vi "Encoder.vi"(11 "Frequency":dbl) -> (1 "Encoder Position (mm)":dbl[](array[numeric]), 2 "RPM":dbl[](array[numeric])=[1.7549382010467513e-60, 1.807415273169756e-52])   [LabVIEW 2021]
uses:
  <vilib>/Analysis/3filter.llb/Filter Passband Type.ctl
  <vilib>/ptbypt/NI_PtbyPt.lvlib
  <vilib>/Analysis/NI_AALBase.lvlib
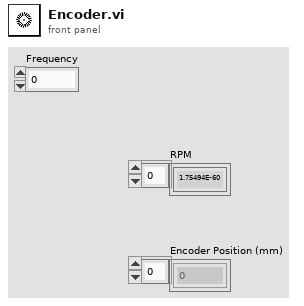
[diagram p1: front panel]
types:
  T1 = typedef "NI_AALBase.lvlib/Filter Passband Type.ctl" = enum32{"Lowpass", "Highpass", "Bandpass", "Bandstop"}
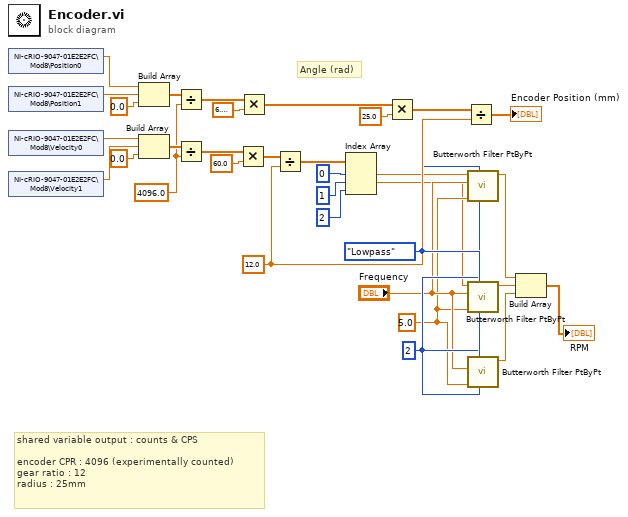
[diagram p0: block diagram]
diagram:
  w19 = 12.0 ("y")
  w23 = 4096.0 ("y")
  w13 = 2 ("order")
  w11 = 5.0 ("low cutoff freq: fl")
  w14 = Filter_Passband_Type."Lowpass" ("filter type")
  # "Angle (rad)"
  # "shared variable output : counts & CPS\n\nencoder CPR : 4096 (experimentally counted)\ngear ratio : 12\nradius : 25mm"
  n1 = shared-variable "NI-cRIO-9047-01E2E2FC\\Mod8\\Position0"() -> (w27:dbl)  [unwired: 1 in, 1 out]
  n2 = shared-variable "NI-cRIO-9047-01E2E2FC\\Mod8\\Position1"() -> (w26:dbl)  [unwired: 1 in, 1 out]
  n3 = shared-variable "NI-cRIO-9047-01E2E2FC\\Mod8\\Velocity0"() -> (w31:dbl)  [unwired: 1 in, 1 out]
  n4 = shared-variable "NI-cRIO-9047-01E2E2FC\\Mod8\\Velocity1"() -> (w30:dbl)  [unwired: 1 in, 1 out]
  n5 = Build Array(w27, w26, 0.0 ("element")) -> (w28:dbl[])
  n6 = Build Array(w31, w30, 0.0 ("element")) -> (w29:dbl[])
  n7 = Divide(x=w28, y=w23) -> (x/y=w25:dbl[])
  n8 = Divide(x=w29, y=w23) -> (x/y=w33:dbl[])
  n9 = Multiply(x=w33, y=60.0) -> (x*y=w18:dbl[])
  n10 = Multiply(x=w25, y=6.283185307179586) -> (x*y=w22:dbl[])
  n11 = Divide(x=w18, y=w19) -> (x/y=w2:dbl[])
  n12 = Index Array(array=w2, index #1=0 ("index"), index #2=1 ("index"), index #3=2 ("index")) -> (element #1=w3:dbl, element #2=w9:dbl)  [unwired: 1 out]
  n13 = Multiply(x=w22, y=25.0) -> (x*y=w20:dbl[])
  n14 = Divide(x=w20, y=w19) -> (x/y=→"Encoder Position (mm)":dbl[])
  n15 = call <vilib>:"Butterworth Filter PtByPt.vi"("order"=w13, "filter type"=w14, "low cutoff freq: fl"=w11, "sampling freq: fs"="Frequency", "x"=w3) -> ("Filtered x"=w5:dbl)  [unwired: 4 in, 1 out]
  n16 = call <vilib>:"Butterworth Filter PtByPt.vi"("order"=w13, "filter type"=w14, "low cutoff freq: fl"=w11, "sampling freq: fs"="Frequency", "x"=w9) -> ("Filtered x"=w6:dbl)  [unwired: 4 in, 1 out]
  n17 = call <vilib>:"Butterworth Filter PtByPt.vi"("order"=w13, "filter type"=w14, "low cutoff freq: fl"=w11, "sampling freq: fs"="Frequency") -> ("Filtered x"=w15:dbl)  [unwired: 5 in, 1 out]
  n18 = Build Array(w5, w6, w15) -> (→"RPM":dbl[])
